vi "Flatten.vi"(6 "Persistence in":refnum<class "IPersist.lvclass">, 7 "Linked List Ref":refnum<data-value>, 8 "error in (no error)":errorcluster, 9 "Indent":i32, 10 "Active Unique ID":string, 11 "Stop Loop in":refnum<class "Stop Loop.lvclass">) -> (0 "error out":errorcluster, 2 "Active Unique ID out":string, 3 "Flattened Test Executive":string[](array[string]), 4 "Persistence out":refnum<class "IPersist.lvclass">, 5 "Linked List Ref out":refnum<data-value>)   [LabVIEW 2019, in "Test Executive.lvlib" / "Stop Loop.lvclass"]
uses:
  <vilib>/gpm_packages/@cs/test-executive/Source/Test Executive/Stop Loop/Stop Loop.lvclass
  <vilib>/gpm_packages/@cs/linked-list/Source/Linked List/ILinkedList/ILinked List.lvclass
  <vilib>/gpm_packages/@cs/persistence/source/IPersist/IPersist.lvclass
  <vilib>/gpm_packages/@cs/test-executive/Source/Test Executive/Executioner/Executioner.lvclass
  <vilib>/gpm_packages/@cs/linked-list/Source/Linked List/Linked List Ref/Linked List Ref.lvclass
  <vilib>/gpm_packages/@cs/linked-list/Source/String Manipulation/String Manipulation.lvlib
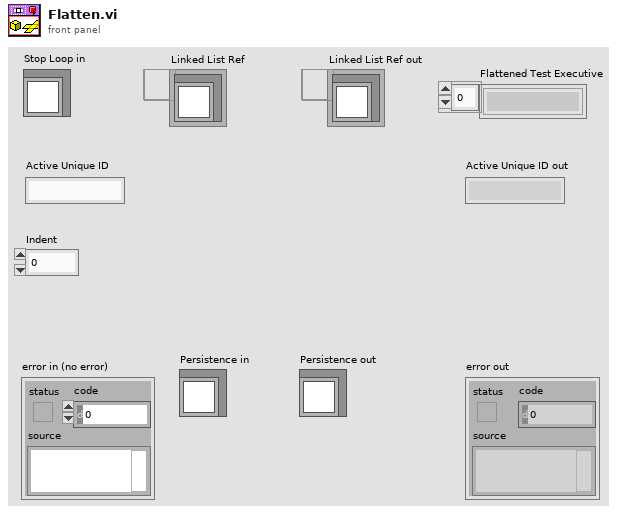
[diagram p1: front panel]
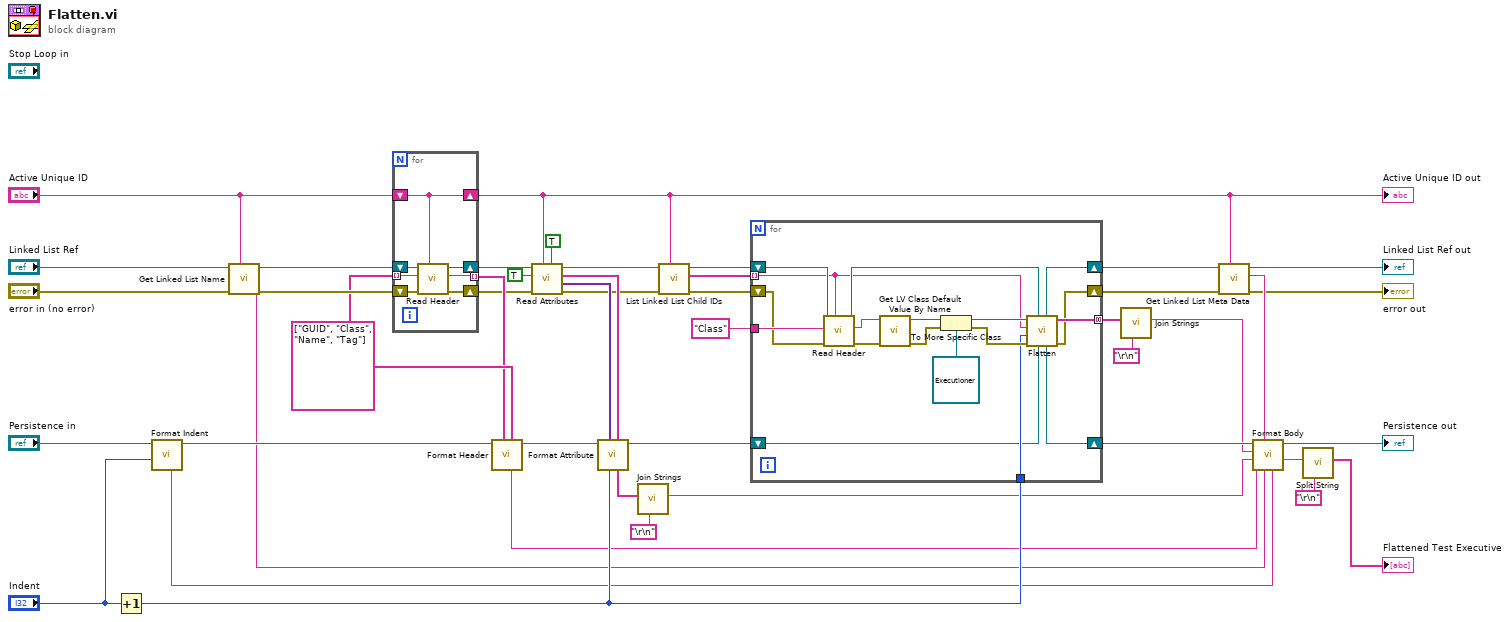
[diagram p0: block diagram]
diagram:
  w42 = string[] ["GUID", "Class", "Name", "Tag"] ("Header Names")
  n1 = Increment(x="Indent") -> (x+1=w23:i32)
  n2 = call-dynamic "Format Indent.vi"("Indent"="Indent", "IPersist in"="Persistence in") -> ("IPersist out"=w43:refnum<class "IPersist.lvclass">, "Indent XML"=w14:string)  [unwired: 7 in, 1 out]
  n3 = call <vilib>:"Get Linked List Name.vi"("Linked List ID"="Active Unique ID", "error in (no error)"="error in (no error)", "Linked List Ref"="Linked List Ref") -> ("error out"=w44:errorcluster, "Linked List Name"=w15:string, "Linked List Ref out"=w45:refnum<data-value>)  [unwired: 5 in, 1 out]
  n4 = for {
    tunnel: w42 -> [w50] mode=indexing
    shift-right: [w51] -> w35
    shift-left: w45 -> [w52]
    tunnel: [w49] -> w41 mode=indexing
    shift-right: [w48] -> w10
    shift-left: "Active Unique ID" -> [w48]
    shift-right: [w46] -> w34
    shift-left: w44 -> [w47]
    n5 = call <vilib>:"Read Header.vi"("Linked List ID"=w48, "error in (no error)"=w47, "Header Name"=w50, "Linked List Ref"=w52) -> ("error out"=w46:errorcluster, "Header Value"=w49:string, "Linked List Ref out"=w51:refnum<data-value>)  [unwired: 4 in, 1 out]
  }
  "Active Unique ID out" <- w10
  n6 = call-dynamic "Format Header.vi"("Name"=w42, "Value"=w41, "IPersist in"=w43) -> ("IPersist out"=w33:refnum<class "IPersist.lvclass">, "Header"=w16:string)  [unwired: 7 in]
  n7 = call <vilib>:"Read Attributes.vi"("Flatten Pointer?"=TRUE, "Linked List ID"=w10, "error in (no error)"=w34, "Include Private?"=TRUE, "Linked List Ref"=w35) -> ("error out"=w31:errorcluster, "Attributes"=w39:variant[], "Attribute Names out"=w38:string[], "Linked List Ref out"=w32:refnum<data-value>)  [unwired: 1 in, 2 out]
  n8 = call-dynamic "Format Attribute.vi"("Attribute Names"=w38, "Indent"=w23, "Attribute Values"=w39, "IPersist in"=w33) -> ("IPersist out"=w24:refnum<class "IPersist.lvclass">, "Attr Strings"=w36:string[])  [unwired: 6 in]
  n9 = call <vilib>:"Join Strings.vi"("Separator (,)"="\r\n", "Strings In"=w36) -> ("String"=w17:string)  [unwired: 9 in]
  n10 = call <vilib>:"List Linked List Child IDs.vi"("Linked List ID"=w10, "error in (no error)"=w31, "Linked List Ref"=w32) -> ("error out"=w26:errorcluster, "Child IDs"=w25:string[], "Linked List Ref out"=w27:refnum<data-value>)  [unwired: 6 in]
  n11 = for {
    shift-right: [w70] -> w13
    shift-left: w27 -> [w69]
    tunnel: w25 -> [w57] mode=indexing
    tunnel: w23 -> [w60]
    shift-right: [w58] -> w19
    shift-left: w24 -> [w59]
    tunnel: [w56] -> w29 mode=concatenating
    shift-right: [w53] -> w12
    shift-left: w26 -> [w54]
    tunnel: "Class" ("Header Name") -> [w55]
    n12 = call <vilib>:"Read Header.vi"("Linked List ID"=w57, "error in (no error)"=w54, "Header Name"=w55, "Linked List Ref"=w69) -> ("error out"=w63:errorcluster, "Header Value"=w64:string, "Linked List Ref out"=w68:refnum<data-value>)  [unwired: 4 in, 1 out]
    n13 = call <vilib>:"Get LV Class Default Value By Name.vi"("error in (no error)"=w63, "class name"=w64) -> ("error out"=w65:errorcluster, "object"=w67:refnum<class>)  [unwired: 8 in]
    n14 = To More Specific Class(target class=refnum<class "Executioner.lvclass"> refnum ("Test Executive.lvlib:Executioner.lvclass"), reference=w67, error in=w65) -> (specific class reference=w62:refnum<class "Executioner.lvclass">, error out=w61:errorcluster)
    n15 = call-dynamic "Flatten.vi"("Persistence in"=w59, "Linked List Ref"=w68, "error in (no error)"=w61, "Indent"=w60, "Active Unique ID"=w57, "Executioner in"=w62) -> ("error out"=w53:errorcluster, "Flattened Test Executive"=w56:string[], "Persistence out"=w58:refnum<class "IPersist.lvclass">, "Linked List Ref out"=w70:refnum<data-value>)  [unwired: 1 in, 1 out]
  }
  n16 = call <vilib>:"Join Strings.vi"("Separator (,)"="\r\n", "Strings In"=w29) -> ("String"=w18:string)  [unwired: 9 in]
  n17 = call <vilib>:"Get Linked List Meta Data.vi"("Linked List ID"=w10, "error in (no error)"=w12, "Linked List Ref"=w13) -> ("error out"=→"error out":errorcluster, "Meta Data"=w22:string, "Linked List Ref out"=→"Linked List Ref out":refnum<data-value>)  [unwired: 5 in, 1 out]
  n18 = call-dynamic "Format Body.vi"("Indent"=w14, "Name"=w15, "Meta Data"=w22, "Header"=w16, "Attributes"=w17, "Body"=w18, "IPersist in"=w19) -> ("String out"=w20:string, "IPersist out"=→"Persistence out":refnum<class "IPersist.lvclass">)  [unwired: 3 in]
  n19 = call <vilib>:"Split String.vi"("Split Pattern"="\r\n", "Input String"=w20) -> ("Split String"=→"Flattened Test Executive":string[])  [unwired: 9 in]
